vi "Initialize.vi"(8 "error in":errorcluster, 11 "Plugin in":refnum<class "Dynamic Channel.lvclass">) -> (0 "error out":errorcluster, 3 "Plugin out":refnum<class "Dynamic Channel.lvclass">)   [LabVIEW 2020, in "Dynamic Channel.lvlib" / "Dynamic Channel.lvclass"]
uses:
  Dynamic Channel.lvclass
  C:/Program Files/National Instruments/LabVIEW 2020/vi.lib/FlexLogger/SDK/PluginSDK.lvlibp/PEFClasses/SDK/Plugin/Plugin.lvclass
  Dynamic Channel.lvclass/Dynamic Channel.ctl
  <vilib>/FlexLogger/SDK/PluginSDK.lvlibp/PEFClasses/SDK/Plugin/ParameterAccess/Write I32.vi
  <vilib>/FlexLogger/SDK/PluginSDK.lvlibp/PEFClasses/SDK/Plugin/Plugin.lvclass
  C:/Program Files/National Instruments/LabVIEW 2020/vi.lib/FlexLogger/SDK/PluginSDK.lvlibp/PEFClasses/SDK/Processing Element/Processing Element.lvclass
  C:/Users/Localization Tester/Documents/LabVIEW Projects/FlexLogger IO Plugins/Dynamic Channel/Dynamic Channel.lvclass
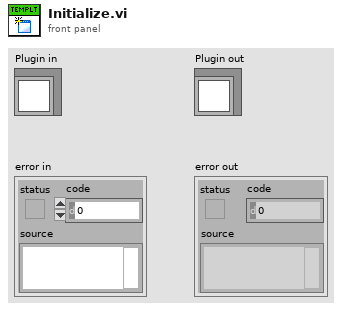
[diagram p1: front panel]
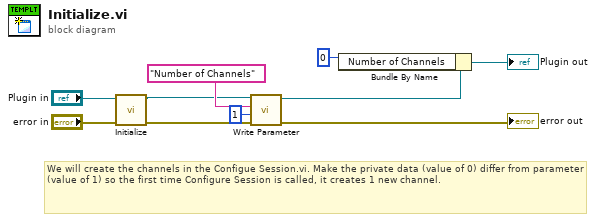
[diagram p0: block diagram]
diagram:
  # "We will create the channels in the Configue Session.vi. Make the private data (value of 0) differ from parameter (value of 1) so the first time Configure Session is called, it creates 1 new channel."
  n1 = call-parent "Initialize.vi"("error in (no error)"="error in", "Plugin in"="Plugin in") -> ("error out"=w6:errorcluster, "Plugin out"=w7:refnum<class "Dynamic Channel.lvclass">)  [unwired: 8 in]
  n2 = call-poly <vilib>:"Write Parameter.vi"("error in (no error)"=w6, "Value"=1, "Name"="Number of Channels", "Plugin in"=w7) -> ("error out"=→"error out":errorcluster, "Plugin out"=w5:refnum<class "Dynamic Channel.lvclass">)  [unwired: 6 in]
  n3 = Bundle By Name(cluster=w5, "Number of Channels"=u32 0) -> (→"Plugin out":refnum<class "Dynamic Channel.lvclass">)
